vi "Multi Graph Toggle.vi"(8 "error in (no error)":errorcluster, 9 "Array":bool[](array[boolean]), 10 "Waveform Chart":refnum<vi>) -> (0 "error out":errorcluster)   [LabVIEW 2023]
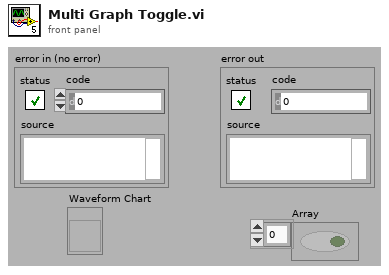
[diagram p1: front panel]
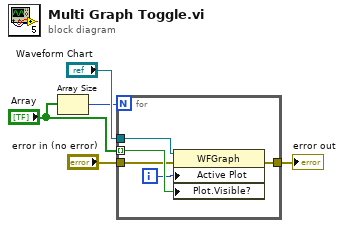
[diagram p0: block diagram]
diagram:
  n1 = Array Size(array="Array") -> (size(s)=w1:i32)
  n2 = for {
    N: w1 -> [_]
    tunnel: "Array" -> [w10] mode=indexing
    tunnel: [w8] -> w5
    tunnel: "error in (no error)" -> [w7]
    tunnel: "Waveform Chart" -> [w6]
    i -> [w9]
    n3 = property on="Property Node" class="WFGraph"(reference=w6, error in=w7, "Active Plot"=w9, "Plot.Visible?"=w10) -> (error out=w8:errorcluster)  [unwired: 1 out]
  }
  "error out" <- w5
